vi "_Create_Message.vi"(9 "Class":path=path "D:/Project/R-Jet/R-Jet/TestVI/Multiple devices Download Tool/Multiple devices Download UI/Multiple devices Download UI/Multiple devices Download UI.lvclass", 10 "Path":path, 11 "Project Path in":path) -> (0 "error out":errorcluster, 2 "Msg.lvclass path":path, 3 "Do path":path)   [LabVIEW 2017]
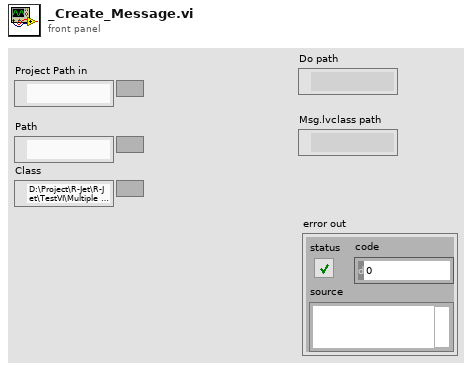
[diagram p1: front panel]
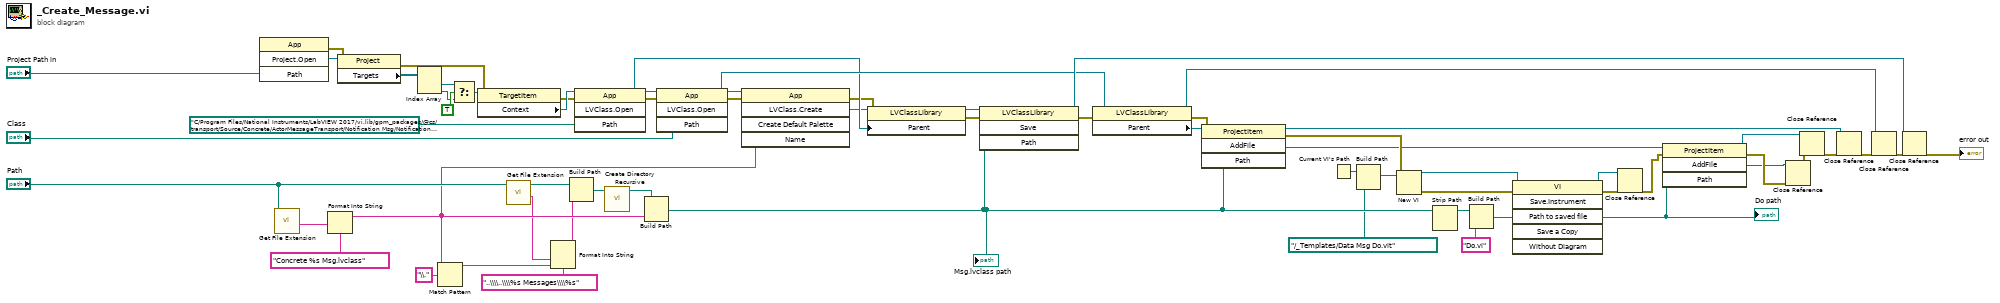
[diagram p0: block diagram]
diagram:
  n1 = invoke class="App" method="Project.Open"("Path"="Project Path in") -> (error out=w7:errorcluster, "Project:Open"=w5:refnum<vi>)  [unwired: 3 in, 2 out]
  n2 = call <vilib>:"Get File Extension.vi"("file"="Path") -> ("filename without extension"=w25:string)  [unwired: 6 in, 4 out]
  n3 = Format Into String(format string="Concrete %s Msg.lvclass", w25) -> (resulting string=w27:string)  [unwired: 2 in, 1 out]
  n4 = property class="Project"(reference=w5, error in=w7) -> (error out=w6:errorcluster, "Targets"=w1:refnum<vi>[])  [unwired: 1 out]
  n5 = Index Array(array=w1) -> (element #1=w2:refnum<vi>, element #2=w3:refnum<vi>)  [unwired: 2 in]
  n6 = Match Pattern(string=w27, regular expression="\\.") -> (before substring=w23:string)  [unwired: 1 in, 3 out]
  n7 = Select(t=w2, s=TRUE ("My Computer?"), f=w3) -> (s? t:f=w4:refnum<vi>)
  n8 = property class="TargetItem"(reference=w4, error in=w6) -> (error out=w8:errorcluster, "Context"=w11:refnum<vi>)  [unwired: 1 out]
  n9 = call <vilib>:"Get File Extension.vi"("file"="Path") -> ("filename without extension"=w19:string, "dup file"=w20:path)  [unwired: 6 in, 3 out]
  n10 = Format Into String(format string="..\\\\..\\\\%s Messages\\\\%s", w19, w23) -> (resulting string=w18:string)  [unwired: 2 in, 1 out]
  n11 = Build Path(base path=w20, name or relative path=w18) -> (appended path=w26:path)
  n12 = invoke class="App" method="LVClass.Open"(reference=w11, error in=w8, "Path"=path "C:/Program Files/National Instruments/LabVIEW 2017/vi.lib/gpm_packages/@cs/transport/Source/Concrete/ActorMessageTransport/Notification Msg/Notification Msg.lvclass") -> (reference out=w12:refnum<vi>, error out=w13:errorcluster, "LVClass.Open"=w43:refnum<vi>)  [unwired: 1 in, 1 out]
  n13 = call <vilib>:"Create Directory Recursive.vi"("directory"=w26) -> ("directory copy"=w24:path)  [unwired: 4 in, 2 out]
  n14 = Build Path(base path=w24, name or relative path=w27) -> (appended path=w57:path)
  "Msg.lvclass path" <- w57
  n15 = invoke class="App" method="LVClass.Open"(reference=w12, error in=w13, "Path"="Class") -> (reference out=w15:refnum<vi>, error out=w16:errorcluster, "LVClass.Open"=w44:refnum<vi>)  [unwired: 1 in, 1 out]
  n16 = invoke class="App" method="LVClass.Create"(reference=w15, error in=w16, "Name"=w27) -> (error out=w29:errorcluster, "LVClass.Create"=w28:refnum<vi>)  [unwired: 2 in, 3 out]
  n17 = property class="LVClassLibrary"(reference=w28, error in=w29, "Parent"=w43) -> (reference out=w32:refnum<vi>, error out=w30:errorcluster)
  n18 = invoke class="LVClassLibrary" method="Save"(reference=w32, error in=w30, "Path"=w57) -> (reference out=w46:refnum<vi>, error out=w31:errorcluster)  [unwired: 1 in, 2 out]
  n19 = property class="LVClassLibrary"(reference=w44, error in=w31) -> (reference out=w45:refnum<vi>, error out=w42:errorcluster, "Parent"=w33:refnum<vi>)
  n20 = invoke class="ProjectItem" method="AddFile"(reference=w33, error in=w42, "Path"=w57) -> (reference out=w52:refnum<vi>, error out=w58:errorcluster, "AddFile"=w41:refnum<vi>)  [unwired: 1 in, 1 out]
  n21 = Current VI's Path() -> (path=w34:path)
  n22 = Build Path(base path=w34, name or relative path=path "../_Templates/Data Msg Do.vit" ("template")) -> (appended path=w35:path)
  n23 = New VI(8:w58, 10:w35) -> (0:w40:errorcluster, 3:w39:refnum<vi>)  [unwired: 5 in]
  n24 = Strip Path(path=w57) -> (stripped path=w37:path)  [unwired: 1 out]
  n25 = Build Path(base path=w37, name or relative path="Do.vi") -> (appended path=w61:path)
  "Do path" <- w61
  n26 = invoke class="VI" method="Save.Instrument"(reference=w39, error in=w40, "Path to saved file"=w61) -> (reference out=w60:refnum<vi>, error out=w59:errorcluster)  [unwired: 3 in, 4 out]
  n27 = Close Reference(reference=w60, error in (no error)=w59) -> (error out=w62:errorcluster)
  n28 = invoke class="ProjectItem" method="AddFile"(reference=w41, error in=w62, "Path"=w61) -> (reference out=w50:refnum<vi>, error out=w56:errorcluster, "AddFile"=w49:refnum<vi>)  [unwired: 1 in, 1 out]
  n29 = Close Reference(reference=w49, error in (no error)=w56) -> (error out=w51:errorcluster)
  n30 = Close Reference(reference=w50, error in (no error)=w51) -> (error out=w48:errorcluster)
  n31 = Close Reference(reference=w52, error in (no error)=w48) -> (error out=w53:errorcluster)
  n32 = Close Reference(reference=w45, error in (no error)=w53) -> (error out=w47:errorcluster)
  n33 = Close Reference(reference=w46, error in (no error)=w47) -> (error out=→"error out":errorcluster)
